vi "Trav_name_to_IP_No.vi"(0 "Trav name":string) -> (1 "VI name":string)   [LabVIEW 2010]
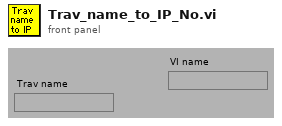
[diagram p1: front panel]
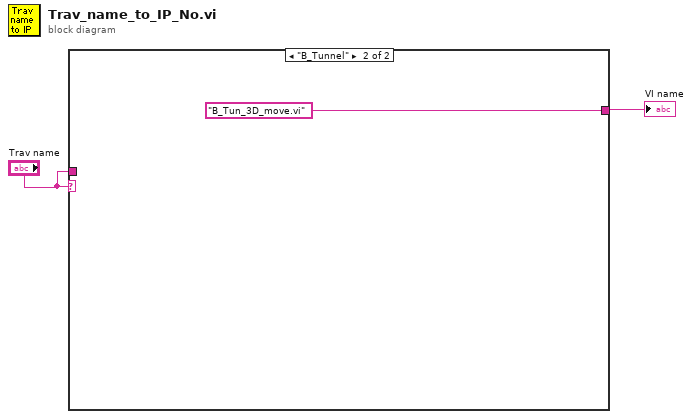
[diagram p0: block diagram]
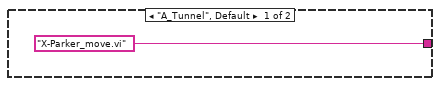
[diagram p2: hidden frame]
diagram:
  n1 = case shown="\"B_Tunnel\"" "Trav name" {
    tunnel: ["X-Parker_move.vi" ("VI name") "B_Tun_3D_move.vi" ("VI name")] -> w2
    tunnel: "Trav name" -> [_ _]
    frame "A_Tunnel", Default {
    }
    frame "B_Tunnel" {
    }
  }
  "VI name" <- w2
